vi "Parsing Error in converting to LabVIEW type.vi"(4 "LV Type":variant, 6 "initial string":string, 7 "JSON":string, 8 "error in (no error)":errorcluster, 9 "Offset past match":i32=-1, 10 "Value start":i32=-1, 11 "State":T1) -> (0 "error out":errorcluster)   [LabVIEW 2020, in "JSONtext.lvlib"]
uses:
  <vilib>/JDP Science/JSONtext/JSONtext.lvlib
  <vilib>/JDP Science/JSONtext/Parsing/Parsing State.ctl
  <vilib>/Utility/Data Type/Type Definitions/Data Type.ctl
  <vilib>/Utility/Data Type/NI_Data Type.lvlib
  <vilib>/JDP Science/JDP Science Common Utilities/JDP Utility.lvlib
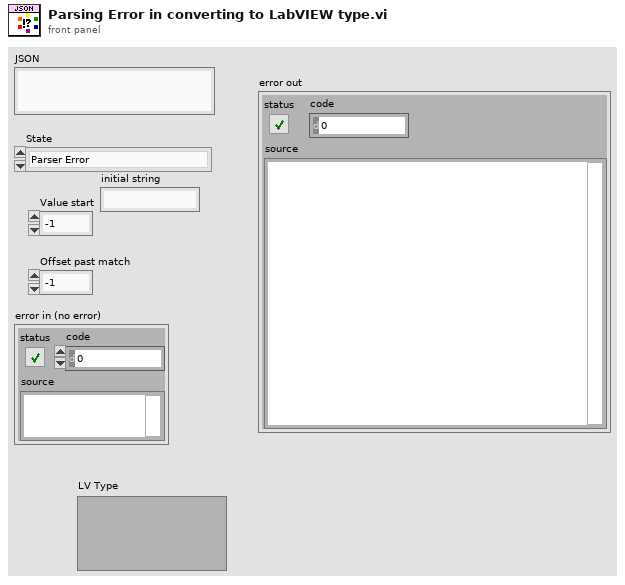
[diagram p1: front panel]
types:
  T1 = typedef "JSONtext.lvlib/Parsing State.ctl" = enum16{"Parser Error", "Object", "Array", "String", "Number/Other", "Leading Whitespace", "Object end", "Array end", "Value end"}
  T2 = typedef "NI_Data Type.lvlib/Data Type.ctl" = enum8{"Invalid Type", "Void", "I8", "I16", "I32", "I64", "U8", "U16", "U32", "U64", "Single Float", "Double Float", "Extended Float", "Single Complex", "Double Complex", "Extended Complex", "Enum U8", "Enum U16", "Enum U32", "Enum U64", "Single Float With Unit", "Double Float With Unit", "Extended Float With Unit", "Single Complex with Unit", "Double Complex with Unit", "Extended Complex with Unit", "Boolean", "String", "Path", "Picture", "Tag", "Array", "Cluster", "Variant", "LV Variant", "Waveform", "Timestamp", "Digital Waveform", "Digital Data", "ExpressData", "Refnum", "External Data", "VI", "Poly VI", "LabVIEW Class Instance", "Fixed Point", "Set Collection", "Map Collection"}
  T3 = typedef "JSONtext.lvlib/JSON Value Type.ctl" = enum16{"Not a JSON Value", "JSON Object", "JSON Array", "String", "Number", "true", "false", "null"}
  T4 = typedef "NI_Data Type.lvlib/Refnum Type.ctl" = enum16{"NotARefnum", "UnknownRefnum", "Generic", "Datalog", "ByteStream", "Device", "Occurence", "TCPNetConnection", "Auto", "Menu", "Imaq", "Hardware", "DataSocket", "Visa", "IVI", "UDPNetConnection", "Notifier", "Queue", "Irda", "EventReg", "DotNet", "UserEvent", "Callback", "UNUSED_EMPTY_POSITION", "BlueToothNetConnection", "LVObjApp", "LVObjVI", "LVObjUnknown", "GenericClass", "UserDefinedRefnumTag", "DataValue", "RT FIFO", "TDMS File", "PythonSessionRefnum"}
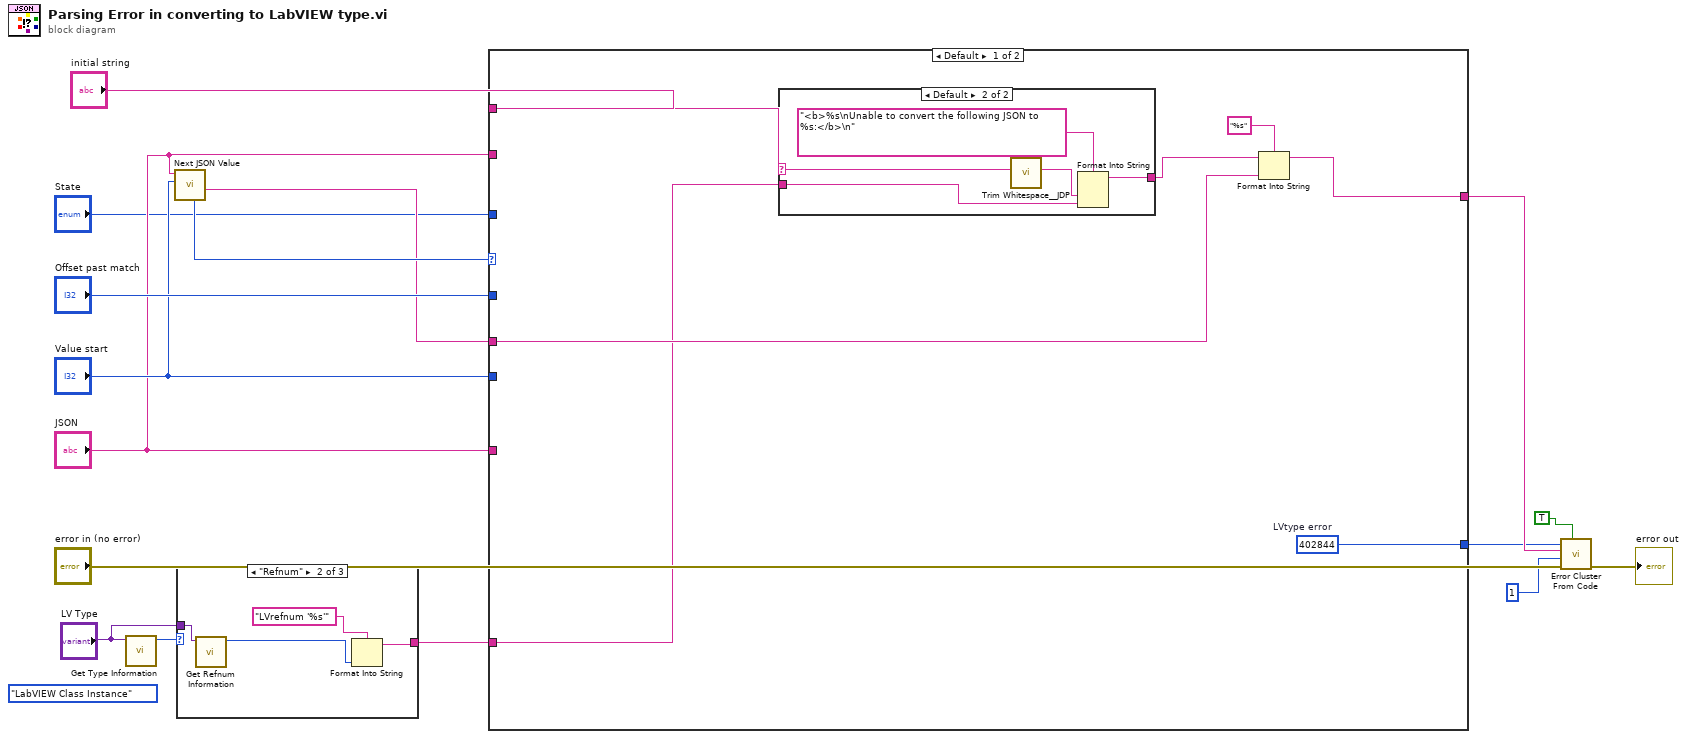
[diagram p0: block diagram]
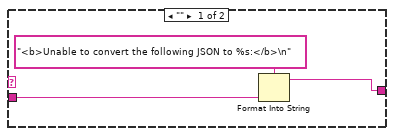
[diagram p2: hidden frame]
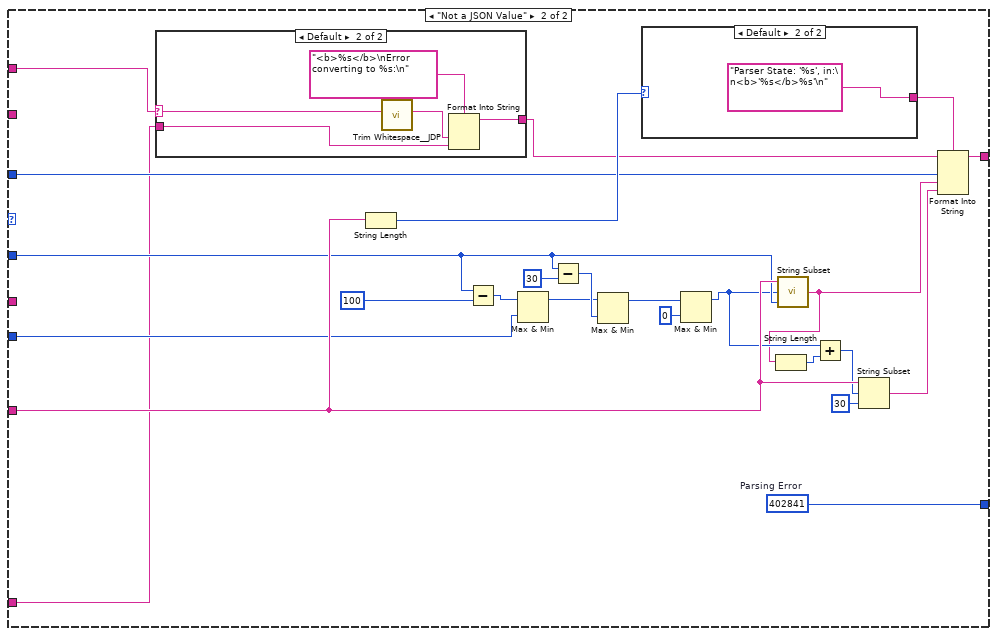
[diagram p3: hidden frame]
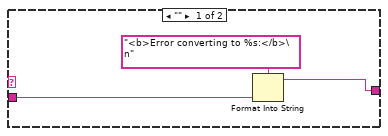
[diagram p4: hidden frame]
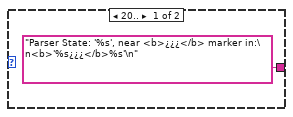
[diagram p5: hidden frame]
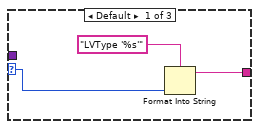
[diagram p6: hidden frame]
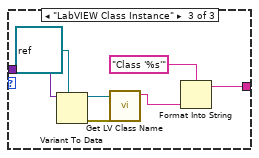
[diagram p7: hidden frame]
diagram:
  (unwired) Data_Type."LabVIEW Class Instance" ("Type")
  n1 = call <vilib>:"Get Type Information.vi"("variant"="LV Type") -> ("type"=w8:T2)  [unwired: 6 in, 4 out]
  n2 = call <vilib>:"Next JSON Value.vi"("Offset"="Value start", "JSON"="JSON") -> ("<JSON>"=w6:string, "JSON Value Type"=w7:T3)  [unwired: 6 in, 2 out]
  n3 = case shown="\"Refnum\"" w8 {
    selector: w8 -> [w19 _ _]
    tunnel: [w18 w22 w26] -> w3
    tunnel: "LV Type" -> [_ w20 w30]
    frame Default {
      n4 = Format Into String(format string="LVType '%s'" ("initial string"), w19) -> (resulting string=w18:string)  [unwired: 2 in, 1 out]
    }
    frame "Refnum" {
      n5 = call <vilib>:"Get Refnum Information.vi"("variant"=w20) -> ("reference type"=w23:T4)  [unwired: 7 in, 3 out]
      n6 = Format Into String(format string="LVrefnum '%s'" ("initial string"), w23) -> (resulting string=w22:string)  [unwired: 2 in, 1 out]
    }
    frame "LabVIEW Class Instance" {
      n7 = Variant To Data(type=refnum<class> refnum ("LabVIEW Object"), Variant=w30) -> (data=w27:refnum<class>, error out=w28:errorcluster)  [unwired: 1 in]
      n8 = call <vilib>:"Get LV Class Name.vi"("error in (no error)"=w28, "object"=w27) -> ("class name"=w25:string)  [unwired: 8 in, 1 out]
      n9 = Format Into String(format string="Class '%s'" ("initial string"), w25) -> (resulting string=w26:string)  [unwired: 2 in, 1 out]
    }
  }
  n10 = case shown="Default" w7 {
    tunnel: [w35 w69] -> w16
    tunnel: "JSON" -> [_ w68]
    tunnel: "Offset past match" -> [_ w67]
    tunnel: [w34 w66] -> w10
    tunnel: "JSON" -> [_ _]
    tunnel: "Value start" -> [_ w50]
    tunnel: w6 -> [w36 _]
    tunnel: "initial string" -> [w31 w46]
    tunnel: "State" -> [_ w49]
    tunnel: w3 -> [w32 w47]
    frame Default {
      w34 = 402844  # LVtype error
      n11 = case shown="Default" w31 {
        selector: w31 -> [_ w45]
        tunnel: [w38 w44] -> w33
        tunnel: w32 -> [w40 w41]
        frame "" {
          n12 = Format Into String(format string="<b>Unable to convert the following JSON to %s:</b>\n", w40) -> (resulting string=w38:string)  [unwired: 2 in, 1 out]
        }
        frame Default {
          n13 = call <vilib>:"Trim Whitespace__JDP.vi"("String in"=w45) -> ("String out"=w42:string)  [unwired: 6 in]
          n14 = Format Into String(format string="<b>%s\nUnable to convert the following JSON to %s:</b>\n", w42, w41) -> (resulting string=w44:string)  [unwired: 2 in, 1 out]
        }
      }
      n15 = Format Into String(format string="%s", initial string=w33, w36) -> (resulting string=w35:string)  [unwired: 1 in, 1 out]
    }
    frame "Not a JSON Value" {
      w66 = 402841  # Parsing Error
      n16 = case shown="Default" w46 {
        selector: w46 -> [_ w77]
        tunnel: [w70 w76] -> w48
        tunnel: w47 -> [w72 w73]
        frame "" {
          n17 = Format Into String(format string="<b>Error converting to %s:</b>\n", w72) -> (resulting string=w70:string)  [unwired: 2 in, 1 out]
        }
        frame Default {
          n18 = call <vilib>:"Trim Whitespace__JDP.vi"("String in"=w77) -> ("String out"=w74:string)  [unwired: 6 in]
          n19 = Format Into String(format string="<b>%s</b>\nError converting to %s:\n", w74, w73) -> (resulting string=w76:string)  [unwired: 2 in, 1 out]
        }
      }
      n20 = String Length(string=w68) -> (length=w51:i32)
      n21 = Subtract(x=w67, y=100) -> (x-y=w63:i32)
      n22 = Max & Min(x=w63, y=w50) -> (max(x,y)=w54:i32)  [unwired: 1 out]
      n23 = Subtract(x=w67, y=30) -> (x-y=w55:i32)
      n24 = Max & Min(x=w54, y=w55) -> (max(x,y)=w53:i32)  [unwired: 1 out]
      n25 = case shown="Default" w51 {
        tunnel: ["Parser State: '%s', near <b>¿¿¿</b> marker in:\n<b>'%s¿¿¿</b>%s'\n" ("format string") "Parser State: '%s', in:\n<b>'%s</b>%s'\n" ("format string")] -> w52
        frame 20.. {
        }
        frame Default {
        }
      }
      n26 = Max & Min(x=w53, y=0) -> (max(x,y)=w61:i32)  [unwired: 1 out]
      n27 = call <vilib>:"String Subset.vi"("Offset past End"=w67, "Start offset"=w61, "JSON"=w68) -> ("substring"=w59:string)  [unwired: 2 in]
      n28 = String Length(string=w59) -> (length=w60:i32)
      n29 = Add(x=w61, y=w60) -> (x+y=w58:i32)
      n30 = String Subset(string=w68, offset (0)=w58, length (rest)=30 ("Offset past End")) -> (substring=w65:string)
      n31 = Format Into String(format string=w52, initial string=w48, w49, w59, w65) -> (resulting string=w69:string)  [unwired: 1 in, 1 out]
    }
  }
  n32 = call <vilib>:"Error Cluster From Code.vi"("show call chain? (True)"=TRUE ("show call chain? (False)"), "error in (no error)"="error in (no error)", "Call Depth"=1, "error message (\"\")"=w16, "error code (402840+)"=w10) -> ("error out"=→"error out":errorcluster)  [unwired: 4 in]
